vi "Chevy_x_DV.vi"(1 "Tn coeffs":dbl[](array[numeric])=[-1.4885517808010453, -0.4725618709636064, 0.4630200814142276, 0.6700741417747852, -0.15642761844645178, -0.10776354749193232, -0.019394804254517988, 0.02480718958930428, 0.011086294796594199, -0.02220834303954161, 0.014194437393199913, 0.00192073719401433, -0.013619305726609358, 0.012299938256651008] format="%.2f", 2 "x":dbl format="%.2f", 3 "end":dbl=7.0 format="%.2f", 4 "start":dbl format="%.2f") -> (0 "f(x)":dbl)   [LabVIEW 2020]
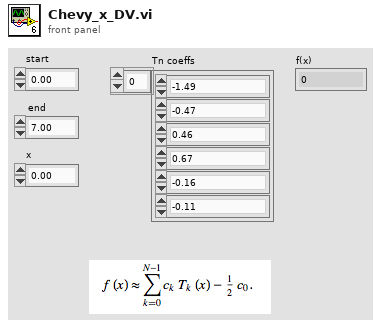
[diagram p1: front panel]
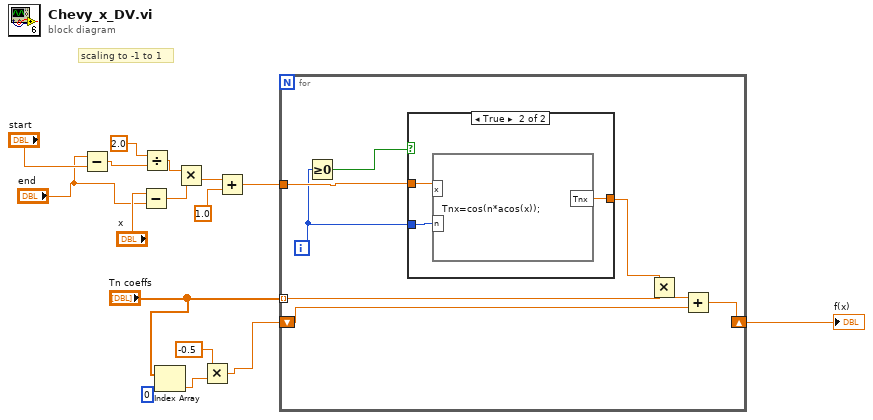
[diagram p0: block diagram]
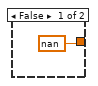
[diagram p2: hidden frame]
diagram:
  # "scaling to -1 to 1"
  n1 = Subtract(x="end", y="start") -> (x-y=w16:dbl)
  n2 = Subtract(x="x", y="end") -> (x-y=w12:dbl)
  n3 = Divide(x=2.0, y=w16) -> (x/y=w14:dbl)
  n4 = Index Array(array="Tn coeffs", index=0) -> (element=w5:dbl)
  n5 = Multiply(x=w14, y=w12) -> (x*y=w11:dbl)
  n6 = Multiply(x=-0.5, y=w5) -> (x*y=w1:dbl)
  n7 = Add(x=w11, y=1.0) -> (x+y=w7:dbl)
  n8 = for {
    tunnel: w7 -> [w24]
    tunnel: "Tn coeffs" -> [w22] mode=indexing
    shift-right: [w18] -> w2
    shift-left: w1 -> [w19]
    i -> [w21]
    n9 = Greater Or Equal To 0?(x=w21) -> (x >= 0?=w17:bool)
    n10 = case shown="True" w17 {
      tunnel: w24 -> [_ w28]
      tunnel: w21 -> [_ w27]
      tunnel: [nan w26] -> w23
      frame False {
      }
      frame True {
        n11 = formula code="Tnx=cos(n*acos(x));"("x"=w28, "n"=w27) -> ("Tnx"=w26:dbl)
      }
    }
    n12 = Multiply(x=w23, y=w22) -> (x*y=w20:dbl)
    n13 = Add(x=w20, y=w19) -> (x+y=w18:dbl)
  }
  "f(x)" <- w2
